vi "Revert Tiles in Set.vi"(9 "Revert? (T)":bool=TRUE, 10 "Set":set{cluster{i32, i32}}(c389), 11 "Board in":T1[][](array[typedef])) -> (2 "Set out":set{cluster{i32, i32}}(c389), 3 "Board out":T1[][](array[typedef]))   [LabVIEW 2019]
doc: "Resets the tiles in the Set to Empty Water if Revert is true. Empties the Set if this action is taken. If Revert is false, no changes are made to the Board or the Set."
uses:
  Tile State.ctl
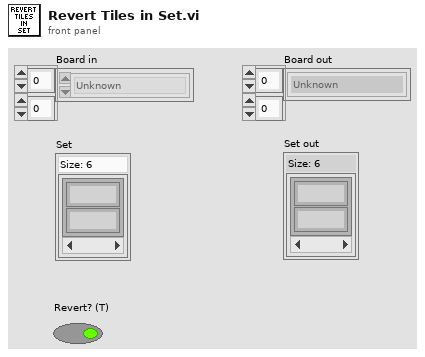
[diagram p1: front panel]
types:
  T1 = typedef "Tile State.ctl" = enum16{"Unknown", "Empty Water", "My Ship (Hidden)", "My Ship (Hit)", "Opponent's Ship (Revealed)", "Oponnent's Ship (Hit)", "Tentative Location"}
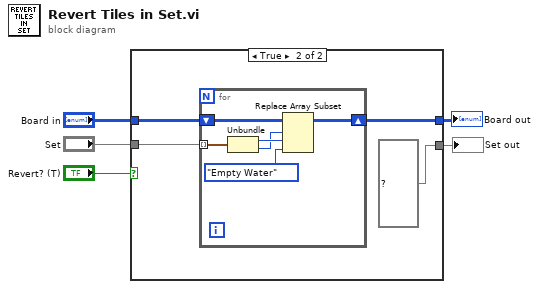
[diagram p0: block diagram]
diagram:
  n1 = case shown="True" "Revert? (T)" {
    tunnel: "Board in" -> [w7 w11]
    tunnel: [w7 w10] -> w3
    tunnel: "Set" -> [w6 w8]
    tunnel: [w6 set{cluster{i32, i32}} {} ("Set out")] -> w1
    frame False {
    }
    frame True {
      n2 = for {
        tunnel: w8 -> [w15] mode=indexing
        shift-right: [w16] -> w10
        shift-left: w11 -> [w17]
        n3 = Unbundle(w15) -> (w14:i32, w13:i32)
        n4 = Replace Array Subset(array=w17, new element=Tile_State."Empty Water" ("new element/subarray"), index (row)=w13, index (col)=w14) -> (w16:T1[][])
      }
    }
  }
  "Board out" <- w3
  "Set out" <- w1
